vi "Perform Draw Scalable Border.vi"(8 "error in (no error)":errorcluster, 11 "Shape in":refnum<class "Shape.lvclass">) -> (0 "error out":errorcluster, 2 "Border out":picture, 3 "Shape out":refnum<class "Shape.lvclass">)   [LabVIEW 2015, in "Shape.lvclass"]
uses:
  Shape.lvclass
  Shape.lvclass/Shape.ctl
  Scalable Border Behavior/Scalable Border Behavior.lvclass
panel:
  # "NOTICE -- YOU MUST LEAVE THIS NOTICE IN PLACE.\n\nCopyright (c) 2017, LIANG LIU Shawn.Liu.cn@gmail.com\nAll rights reserved.\n\nRedistribution and use in source and binary forms, with or without modification, are permitted provided that the following conditions are met:\n-Redistributions of source code must retain the above copyright notice, this list of conditions and the following disclaimer.\n-Redistributions in binary form must reproduce the above copyright notice, this list of conditions and the following disclaimer in the documentation and/or other materials provided with the distribution.\n-Neither the name of the eLp nor the names of its contributors may be used to endorse or promote products derived from this software without specific prior written permission.\n\nTHIS SOFTWARE IS PROVIDED BY THE COPYRIGHT HOLDERS AND CONTRIBUTORS \"AS IS\" AND ANY EXPRESS OR IMPLIED WARRANTIES, INCLUDING, BUT NOT LIMITED TO, THE IMPLIED WARRANTIES OF MERCHANTABILITY AND FITNESS FOR A PARTICULAR PURPOSE ARE DISCLAIMED. IN NO EVENT SHALL THE COPYRIGHT HOLDER OR CONTRIBUTORS BE LIABLE FOR ANY DIRECT, INDIRECT, INCIDENTAL, SPECIAL, EXEMPLARY, OR CONSEQUENTIAL DAMAGES (INCLUDING, BUT NOT LIMITED TO, PROCUREMENT OF SUBSTITUTE GOODS OR SERVICES; LOSS OF USE, DATA, OR PROFITS; OR BUSINESS INTERRUPTION) HOWEVER CAUSED AND ON ANY THEORY OF LIABILITY, WHETHER IN CONTRACT, STRICT LIABILITY, OR TORT (INCLUDING NEGLIGENCE OR OTHERWISE) ARISING IN ANY WAY OUT OF THE USE OF THIS SOFTWARE, EVEN IF ADVISED OF THE POSSIBILITY OF SUCH DAMAGE."
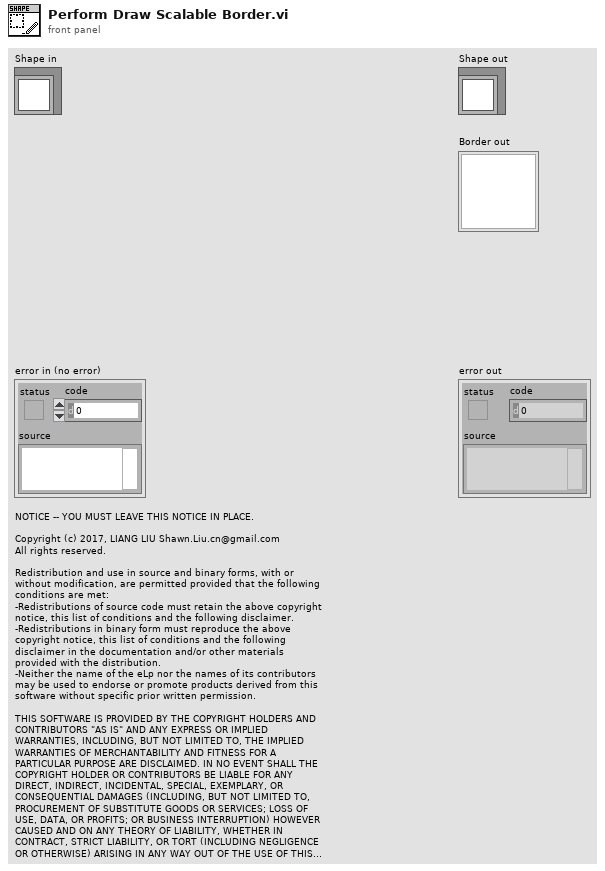
[diagram p1: front panel]
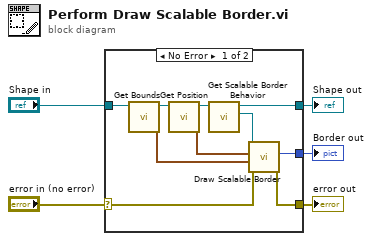
[diagram p0: block diagram]
diagram:
  n1 = case shown="No Error" "error in (no error)" {
    selector: "error in (no error)" -> [w6 w17]
    tunnel: "Shape in" -> [w15 w16]
    tunnel: [w14 w16] -> w4
    tunnel: [w8 _] -> w2
    tunnel: [w7 w17] -> w1
    frame No Error {
      n2 = call "Get Bounds.vi"("Shape in"=w15) -> ("Bounds"=w9:cluster{"Width":u32, "Height":u32}, "Shape out"=w12:refnum<class "Shape.lvclass">)  [unwired: 9 in]
      n3 = call "Get Position.vi"("Shape in"=w12) -> ("Position"=w10:cluster{"Left":i32, "Top":i32}, "Shape out"=w13:refnum<class "Shape.lvclass">)  [unwired: 9 in]
      n4 = call "Get Scalable Border Behavior.vi"("Shape in"=w13) -> ("Scalable Border Behavior"=w11:refnum<class "Scalable Border Behavior.lvclass">, "Shape out"=w14:refnum<class "Shape.lvclass">)  [unwired: 9 in]
      n5 = call-dynamic "Draw Scalable Border.vi"("error in (no error)"=w6, "Bounds"=w9, "Position"=w10, "Scalable Border Behavior in"=w11) -> ("error out"=w7:errorcluster, "Border out"=w8:picture)  [unwired: 5 in, 1 out]
    }
    frame Error {
    }
  }
  "error out" <- w1
  "Shape out" <- w4
  "Border out" <- w2
